vi "createImage.vi"(7 "Upside down":bool, 8 "error in (no error)":errorcluster, 11 "Array":u8[](array[numeric])) -> (0 "error out":errorcluster, 3 "image data":T1)   [LabVIEW 2018]
uses:
  <vilib>/picture/picture.llb/imagedata.ctl
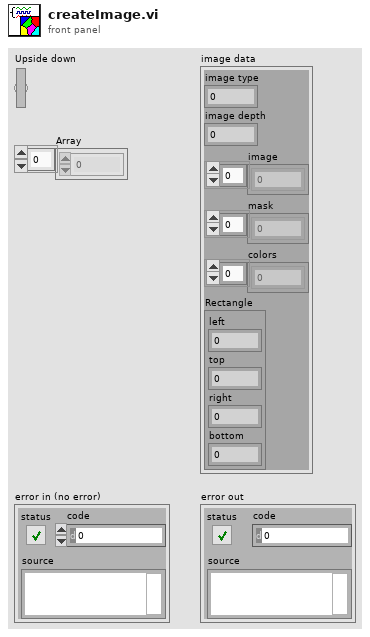
[diagram p1: front panel]
types:
  T1 = typedef "imagedata.ctl" = cluster{"image type":i32, "image depth":i32, "image":u8[], "mask":u8[], "colors":u32[], "Rectangle":cluster{"left":i16, "top":i16, "right":i16, "bottom":i16}}
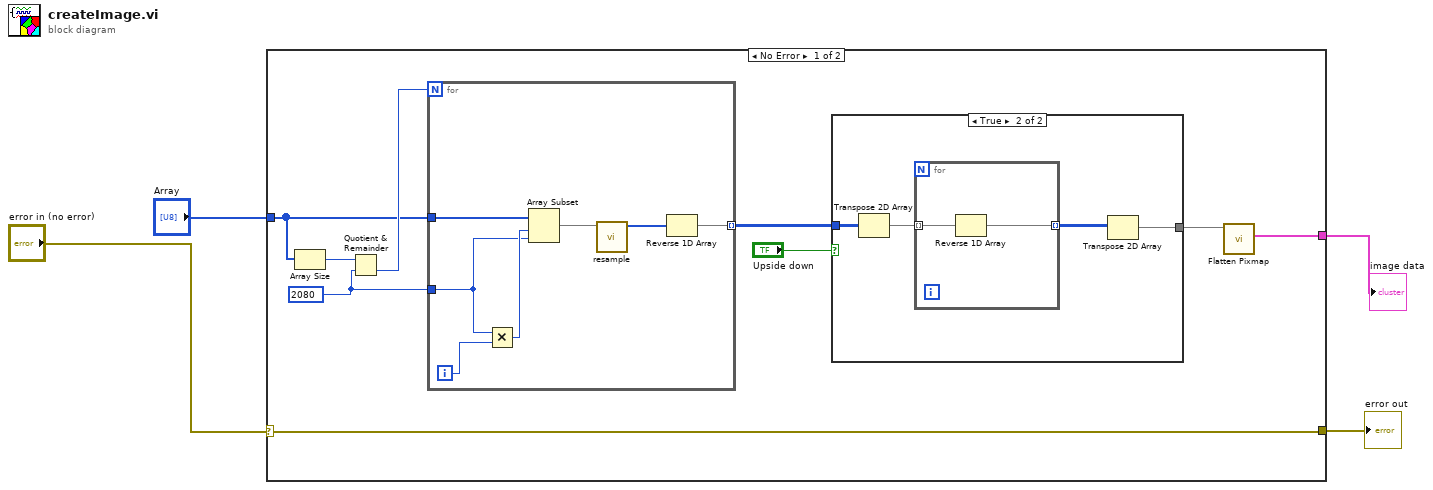
[diagram p0: block diagram]
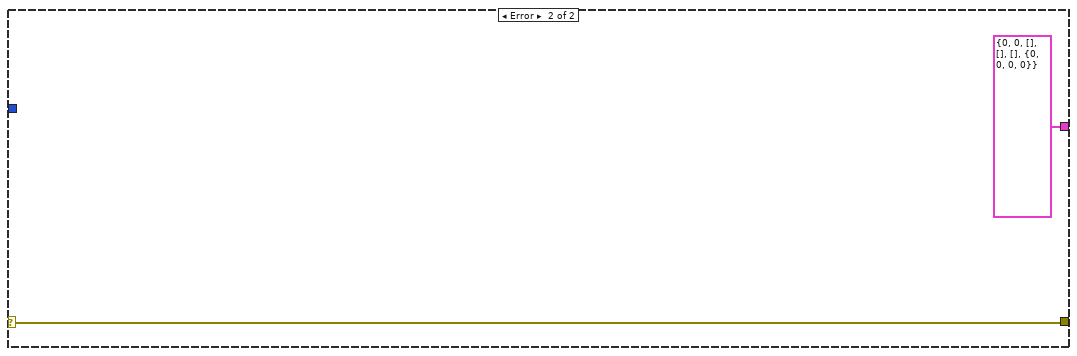
[diagram p3: hidden frame]
diagram:
  n1 = case shown="No Error" "error in (no error)" {
    selector: "error in (no error)" -> [w5 w28]
    tunnel: [w10 T1 {"image type"=0, "image depth"=0, "image"=[], "mask"=[], "colors"=[], "Rectangle"={"left"=0, "top"=0, "right"=0, "bottom"=0}} ("image data")] -> w1
    tunnel: "Array" -> [w6 _]
    tunnel: [w5 w28] -> w4
    frame No Error {
      w11 = 2080 ("y")
      n2 = Array Size(array=w6) -> (size(s)=w13:i32)
      n3 = Quotient & Remainder(x=w13, y=w11) -> (floor(x/y)=w12:i32)  [unwired: 1 out]
      n4 = for {
        N: w12 -> [_]
        tunnel: w6 -> [w27]
        tunnel: [w23] -> w8 mode=indexing
        tunnel: w11 -> [w24]
        i -> [w26]
        n5 = Multiply(x=w24, y=w26) -> (x*y=w25:i32)
        n6 = Array Subset(array=w27, index=w25, length=w24) -> (w22:u8[])
        n7 = call "resample.vi"("Array in"=w22) -> ("Array out"=w21:u32[])  [unwired: 10 in]
        n8 = Reverse 1D Array(array=w21) -> (reversed array=w23:u32[])
      }
      n9 = case shown="True" "Upside down" {
        tunnel: w8 -> [w14 w16]
        tunnel: [w14 w15] -> w7
        frame False {
        }
        frame True {
          n10 = Transpose 2D Array(2D array=w16) -> (transposed array=w18:u32[][])
          n11 = for {
            tunnel: w18 -> [w20] mode=indexing
            tunnel: [w19] -> w17 mode=indexing
            n12 = Reverse 1D Array(array=w20) -> (reversed array=w19:u32[])
          }
          n13 = Transpose 2D Array(2D array=w17) -> (transposed array=w15:u32[][])
        }
      }
      n14 = call <vilib>:"Flatten Pixmap.vi"("24-bit pixmap"=w7) -> ("image data"=w10:T1)  [unwired: 10 in]
    }
    frame Error {
    }
  }
  "error out" <- w4
  "image data" <- w1
